vi "Create Thread Network.vi"(8 "error in (no error)":errorcluster, 11 "Rocom Tests in":refnum<class "Rocom Tests.lvclass">) -> (0 "error out":errorcluster, 3 "Rocom Tests out":refnum<class "Rocom Tests.lvclass">)   [LabVIEW 2015, in "Rocom Tests.lvclass"]
uses:
  Rocom Tests.lvclass
  Classes/Manufacturing Test/Class/SC Manufacturing Test.lvclass
  <vilib>/Cree, Inc/Cree Test Framework/Classes/Base Objects/Base Class/Base Class/Base Class.lvclass
  Classes/Application/Class/Application.lvclass
  Classes/Test Recipe/Class/Test Recipe.lvclass
  Test Class/Test Class.lvclass
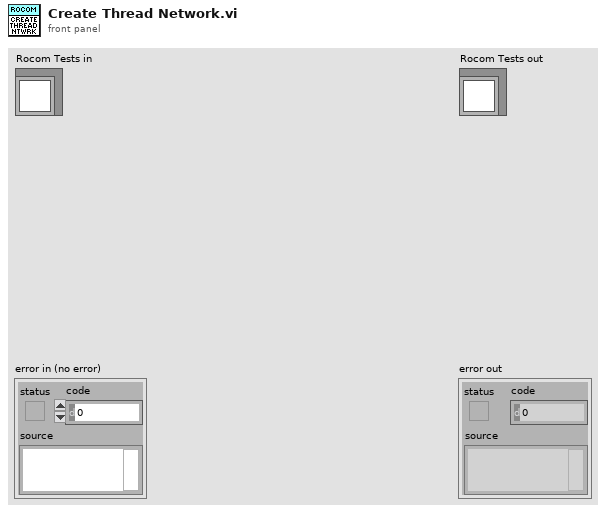
[diagram p1: front panel]
types:
  T1 = typedef "Application.lvlib/App Properties.lvclass/Class Properties -- Cluster.ctl" = cluster{"UUT Info":T2[], "Test Information":refnum<vi>, "Test Complete Event":refnum<user-event>, "Shop Floor System":refnum<class "Shop Floor System.lvclass">, "Gold Board":refnum<class "Golden Board.lvclass">, "Test Recipe":refnum<class "Test Recipe.lvclass">, "Instruments":refnum<class "Instrument.lvclass">[], "Mode":T3, "Test Results":cluster{"Pass":bool[], "Fail Codes":string[]}, "Station Config":refnum<class "Station Config.lvclass">}
  T2 = typedef "Application.lvlib/App Properties.lvclass/UUT Reference -- Cluster.ctl" = cluster{"Serial Number Reference":refnum<vi>, "Status Message Reference":refnum<vi>}
  T3 = typedef "Application.lvlib/Application.lvclass/Op Mode -- Enum.ctl" = u16
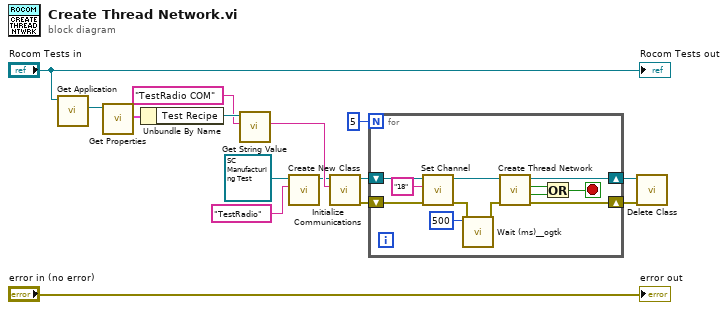
[diagram p0: block diagram]
diagram:
  n1 = call "Get Application.vi"("Test Class in"="Rocom Tests in") -> ("Application.lvlib:Application.lvclass"=w1:refnum<class "Application.lvclass">)  [unwired: 9 in, 1 out]
  n2 = call "Get Properties.vi"("Acrobat Template in"=w1) -> ("Class Properties"=w12:T1)  [unwired: 8 in, 2 out]
  n3 = Unbundle By Name(w12) -> ("Test Recipe"=w13:refnum<class "Test Recipe.lvclass">)
  n4 = call "Get String Value.vi"("Name"="TestRadio COM", "Test Recipe in"=w13) -> ("Value"=w14:string)  [unwired: 7 in, 2 out]
  n5 = call <vilib>:"Create New Class.vi"("Name"="TestRadio", "Base Class in"=refnum<class "SC Manufacturing Test.lvclass"> refnum ("SC Manufacturing Test.lvlib:SC Manufacturing Test.lvclass")) -> ("Base Class out"=w6:refnum<class "SC Manufacturing Test.lvclass">)  [unwired: 8 in, 1 out]
  n6 = call "Initialize Communications.vi"("COM Port"=w14, "Acrobat Template in"=w6) -> ("error out"=w8:errorcluster, "Acrobat Template out"=w7:refnum<class "SC Manufacturing Test.lvclass">)  [unwired: 8 in]
  n7 = for {
    N: 5 -> [_]
    shift-right: [w23] -> w9
    shift-left: w7 -> [w27]
    shift-right: [w22] -> w10
    shift-left: w8 -> [w26]
    stop <- w16 stop-if-true
    n8 = call "Set Channel.vi"("error in (no error)"=w26, "Channel"="18", "Acrobat Template in"=w27) -> ("error out"=w19:errorcluster, "Acrobat Template out"=w25:refnum<class "SC Manufacturing Test.lvclass">)  [unwired: 7 in]
    n9 = call <userlib>:"Wait (ms)__ogtk.vi"("error in (no error)"=w19, "milliseconds to wait"=u32 500) -> ("error out"=w18:errorcluster)  [unwired: 8 in, 1 out]
    n10 = call "Create Thread Network.vi"("error in (no error)"=w18, "Acrobat Template in"=w25) -> ("error out"=w22:errorcluster, "Already Joined"=w21:bool, "Created"=w20:bool, "Acrobat Template out"=w23:refnum<class "SC Manufacturing Test.lvclass">)  [unwired: 6 in]
    n11 = Or(x=w20, y=w21) -> (x .or. y?=w16:bool)
  }
  n12 = call <vilib>:"Delete Class.vi"("error in (no error)"=w10, "Base Class in"=w9) -> ()  [unwired: 8 in, 2 out]
  "error out" <- "error in (no error)"
  "Rocom Tests out" <- "Rocom Tests in"
